vi "Send Slave Node-ID Selected.vi"(7 "Message Priority (Normal)":T1=enum."Normal", 8 "error in (no error)":errorcluster, 10 "Valid?":bool, 11 "Message Enqueuer":refnum<class "Message Enqueuer.lvclass">) -> (0 "error out":errorcluster, 3 "Message Enqueuer out":refnum<class "Message Enqueuer.lvclass">)   [LabVIEW 2024, in "Home.lvlib" / "Slave Node-ID Selected Msg.lvclass"]
doc: "This VI sends the message to an actor."
uses:
  Slave Node-ID Selected Msg.lvclass
  <vilib>/ActorFramework/Message Enqueuer/Message Enqueuer.lvclass
  <vilib>/ActorFramework/Message Enqueuer/Message Priority.ctl
  C:/Program Files/National Instruments/LabVIEW 2024/vi.lib/ActorFramework/Message/Message.lvclass
  Slave Node-ID Selected Msg.lvclass/Slave Node-ID Selected Msg.ctl
  <vilib>/ActorFramework/Message Enqueuer/Message Enqueuer.lvclass/Message Enqueuer.ctl
  <vilib>/Utility/LVClass/Get LV Class Name.vi
  <resource>/AFDebug/Generate Trace for Message.vi
  <vilib>/ActorFramework/Message Priority Queue/Priority Enqueue.vi
  D:/git/CANopen-XNET/Example/Home Messages/Slave Node-ID Selected Msg/Slave Node-ID Selected Msg.lvclass
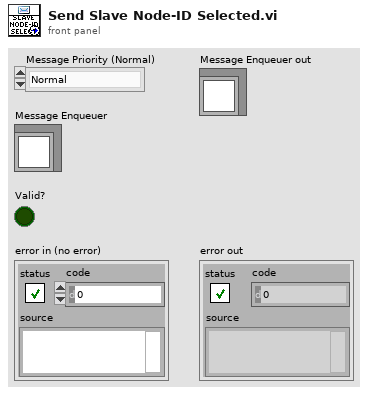
[diagram p1: front panel]
types:
  T1 = typedef "Actor Framework.lvlib/Message Enqueuer.lvclass/Message Priority.ctl" = enum16{"Low", "Normal", "High"}
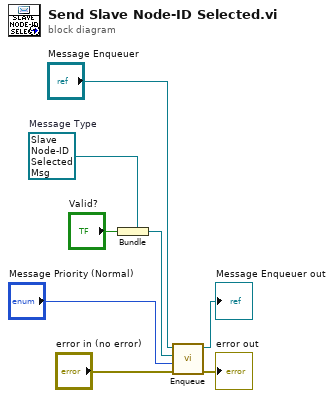
[diagram p0: block diagram]
diagram:
  w5 = refnum<class "Slave Node-ID Selected Msg.lvclass"> refnum  # Message Type
  n1 = Bundle(cluster=w5, "Valid?") -> (w4:refnum<class "Slave Node-ID Selected Msg.lvclass">)
  n2 = call <vilib>:"Enqueue.vi"("error in (no error)"="error in (no error)", "Message Priority (Normal)"="Message Priority (Normal)", "Message"=w4, "Message Enqueuer in"="Message Enqueuer") -> ("error out"=→"error out":errorcluster, "Message Enqueuer in"=→"Message Enqueuer out":refnum<class "Message Enqueuer.lvclass">)  [unwired: 6 in]
